vi "LMData_terminate.vi"(8 "error in (no error)":errorcluster, 11 "LMData in":refnum<class "LMData.lvclass">) -> (0 "error out":errorcluster, 3 "LMData out":refnum<class "LMData.lvclass">)   [LabVIEW 2017, in "LMData.lvclass"]
uses:
  LMData.lvclass
  LMData.lvclass/LMData.ctl
  <instrlib>/Agilent 34401/Agilent 34401.lvlib
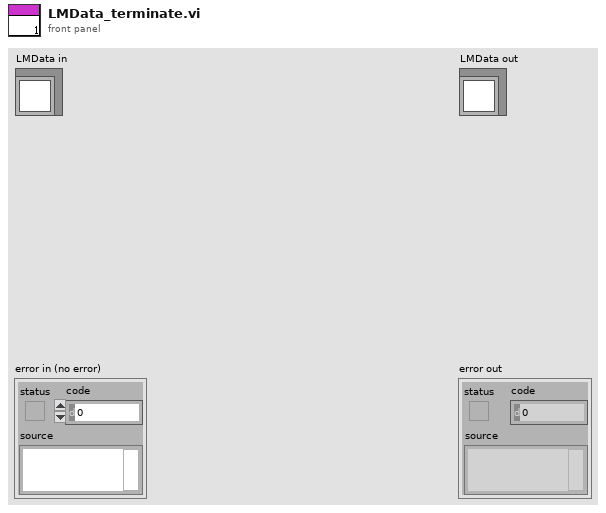
[diagram p1: front panel]
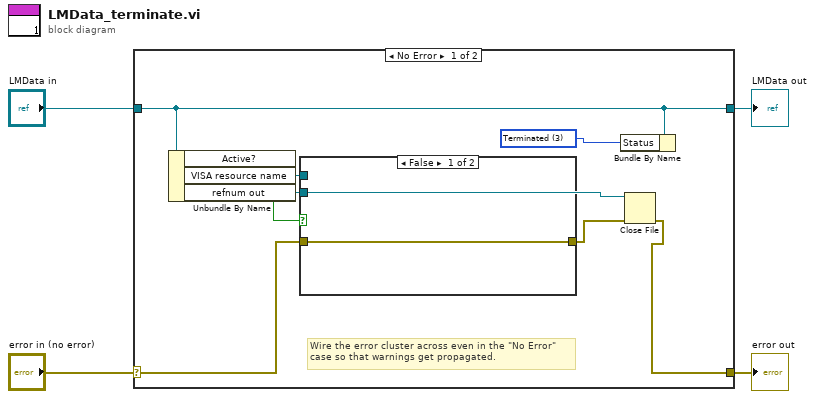
[diagram p0: block diagram]
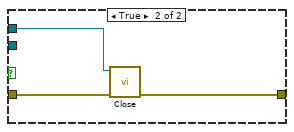
[diagram p2: hidden frame]
diagram:
  n1 = case shown="No Error" "error in (no error)" {
    selector: "error in (no error)" -> [w10 w18]
    tunnel: [w7 w18] -> w3
    tunnel: [w6 w17] -> w1
    tunnel: "LMData in" -> [w6 w17]
    frame No Error {
      w5 = u16 3 items=["Initialized", "Waiting", "Measuring", "Terminated"] ("Status")
      # "Wire the error cluster across even in the \"No Error\"\ncase so that warnings get propagated."
      n2 = Unbundle By Name(w6) -> ("Active?"=w12:bool, "VISA resource name"=w11:refnum<visa-resource-name>, "refnum out"=w9:refnum<file>)
      n3 = case shown="False" w12 {
        tunnel: w11 -> [_ w16]
        tunnel: w10 -> [w13 w15]
        tunnel: [w13 w14] -> w8
        tunnel: w9 -> [_ _]
        frame False {
        }
        frame True {
          n4 = call <instrlib>:"Close.vi"("error in (no error)"=w15, "VISA resource name"=w16) -> ("error out"=w14:errorcluster)  [unwired: 9 in]
        }
      }
      n5 = Bundle By Name(cluster=w6, "Status"=w5) -> ()  [unwired: 1 out]
      n6 = Close File(refnum=w9, error in=w8) -> (error out=w7:errorcluster)  [unwired: 1 out]
    }
    frame Error {
    }
  }
  "error out" <- w3
  "LMData out" <- w1
